vi "GetImgIndexbyChannelInfo.vi"(11 "Channel Info":string) -> (3 "Img Index for Mode Functionality":u16)   [LabVIEW 2021, in "myRIOMetaDataObj.lvclass"]
uses:
  myRIOMetaDataObj.lvclass
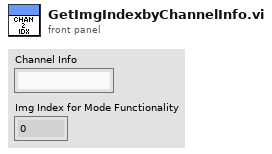
[diagram p1: front panel]
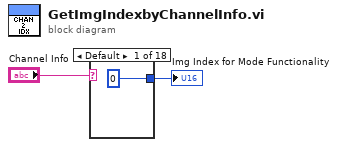
[diagram p0: block diagram]
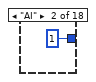
[diagram p2: hidden frame]
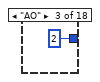
[diagram p3: hidden frame]
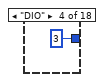
[diagram p4: hidden frame]
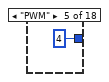
[diagram p5: hidden frame]
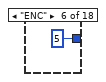
[diagram p6: hidden frame]
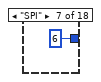
[diagram p7: hidden frame]
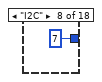
[diagram p8: hidden frame]
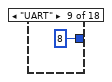
[diagram p9: hidden frame]
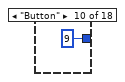
[diagram p10: hidden frame]
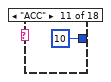
[diagram p11: hidden frame]
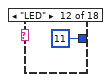
[diagram p12: hidden frame]
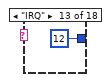
[diagram p13: hidden frame]
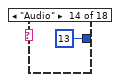
[diagram p14: hidden frame]
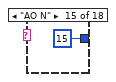
[diagram p15: hidden frame]
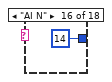
[diagram p16: hidden frame]
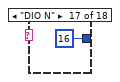
[diagram p17: hidden frame]
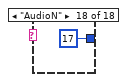
[diagram p18: hidden frame]
diagram:
  n1 = case shown="Default" "Channel Info" {
    tunnel: [u16 0 ("Img Index for Mode Functionality") u16 1 ("Img Index for Mode Functionality") u16 2 ("Img Index for Mode Functionality") u16 3 ("Img Index for Mode Functionality") u16 4 ("Img Index for Mode Functionality") u16 5 ("Img Index for Mode Functionality") u16 6 ("Img Index for Mode Functionality") u16 7 ("Img Index for Mode Functionality") u16 8 ("Img Index for Mode Functionality") u16 9 ("Img Index for Mode Functionality") u16 10 ("Img Index for Mode Functionality") u16 11 ("Img Index for Mode Functionality") u16 12 ("Img Index for Mode Functionality") u16 13 ("Img Index for Mode Functionality") u16 15 ("Img Index for Mode Functionality") u16 14 ("Img Index for Mode Functionality") u16 16 ("Img Index for Mode Functionality") u16 17 ("Img Index for Mode Functionality")] -> w1
    frame Default {
    }
    frame "AI" {
    }
    frame "AO" {
    }
    frame "DIO" {
    }
    frame "PWM" {
    }
    frame "ENC" {
    }
    frame "SPI" {
    }
    frame "I2C" {
    }
    frame "UART" {
    }
    frame "Button" {
    }
    frame "ACC" {
    }
    frame "LED" {
    }
    frame "IRQ" {
    }
    frame "Audio" {
    }
    frame "AO N" {
    }
    frame "AI N" {
    }
    frame "DIO N" {
    }
    frame "AudioN" {
    }
  }
  "Img Index for Mode Functionality" <- w1
